vi "Wait for Operation Complete.vi"(8 "error in (no error)":errorcluster, 10 "Maximum Time (10000mSec)":i32=10000 min=0, 11 "VISA resource name":refnum<visa-resource-name>) -> (0 "error out":errorcluster, 3 "VISA resource name out":refnum<visa-resource-name>)   [LabVIEW 2023, in "Anritsu Signal Analyzer Series.lvlib"]
doc: "Wait for Operation Complete."
uses:
  Anritsu Signal Analyzer Series.lvlib
panel:
  # "mSec"
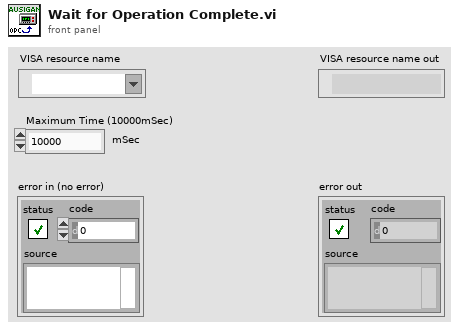
[diagram p1: front panel]
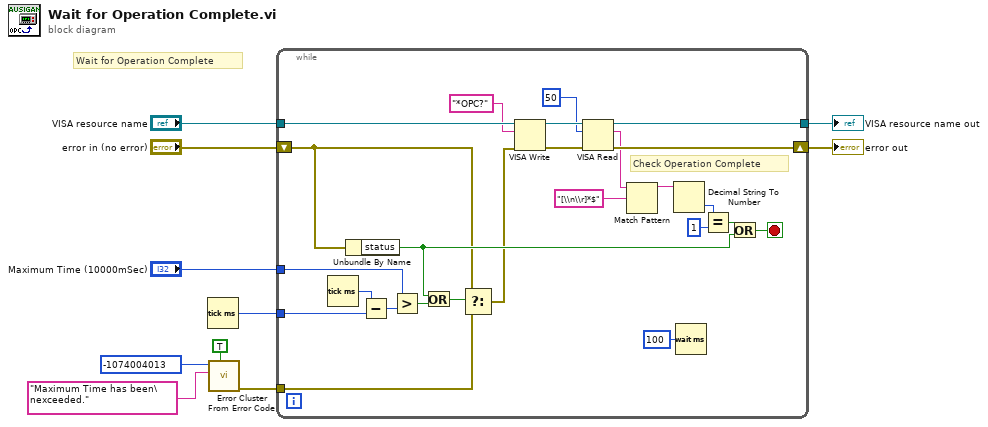
[diagram p0: block diagram]
diagram:
  # "Wait for Operation Complete"
  n1 = Tick Count (ms)() -> (millisecond timer value=w4:u32)
  n2 = call <vilib>:"Error Cluster From Error Code.vi"("show call chain? (False)"=TRUE, "error message (\"\")"="Maximum Time has been\nexceeded." ("error message (\"\")"), "error code (0)"=-1074004013) -> ("error out"=w3:errorcluster)  [unwired: 6 in]
  n3 = while {
    tunnel: "VISA resource name" -> [w35]
    tunnel: [w34] -> w10
    shift-right: [w33] -> w9
    shift-left: "error in (no error)" -> [w13]
    tunnel: "Maximum Time (10000mSec)" -> [w18]
    tunnel: w4 -> [w17]
    tunnel: w3 -> [w11]
    stop <- w14 stop-if-true
    # "Check Operation Complete"
    n4 = Tick Count (ms)() -> (millisecond timer value=w22:u32)
    n5 = Unbundle By Name(w13) -> ("status"=w15:bool)
    n6 = Subtract(x=w22, y=w17) -> (x-y=w21:u32)
    n7 = Greater?(x=w18, y=w21) -> (0:w19:bool)
    n8 = Or(x=w15, y=w19) -> (x .or. y?=w20:bool)
    n9 = Select(t=w13, s=w20, f=w11) -> (s? t:f=w12:errorcluster)
    n10 = VISA Write(VISA resource name=w35, write buffer="*OPC?", error in (no error)=w12) -> (VISA resource name out=w32:refnum<visa-resource-name>, error out=w31:errorcluster)  [unwired: 1 out]
    n11 = VISA Read(VISA resource name=w32, byte count=u32 50 ("byte count (0)"), error in (no error)=w31) -> (VISA resource name out=w34:refnum<visa-resource-name>, read buffer=w29:string, error out=w33:errorcluster)  [unwired: 1 out]
    n12 = Match Pattern(string=w29, regular expression="[\\n\\r]*$") -> (before substring=w25:string)  [unwired: 1 in, 3 out]
    n13 = Decimal String To Number(string=w25) -> (number=w24:i32)  [unwired: 2 in, 1 out]
    n14 = Wait (ms)(milliseconds to wait=u32 100 ("ミリ秒待機時間")) -> ()  [unwired: 1 out]
    n15 = Equal?(x=w24, y=1) -> (x = y?=w16:bool)
    n16 = Or(x=w16, y=w15) -> (x .or. y?=w14:bool)
  }
  "VISA resource name out" <- w10
  "error out" <- w9
